vi "New motor Control integrated remodeled PID revisit.vi"(0 "States":enum16{"RESET ENCODER", "WRITE", "READ", "INIT"}(ring), 1 "Target Speed":T2 {"wTargetSpeed" scale=-1.0..1.0; "yTargetSpeed" scale=-1.0..1.0; "xTargetSpeed" scale=-1.0..1.0}, 3 "Error in":errorcluster, 4 "Boolean":bool=TRUE) -> (5 "Speed and distance cluster":T1, 6 "Error out":errorcluster)   [LabVIEW 2018]
uses:
  <vilib>/addons/control/pid/pid.llb/PID (DBL).vi
  <vilib>/addons/control/pid/NI_PID_pid.lvlib
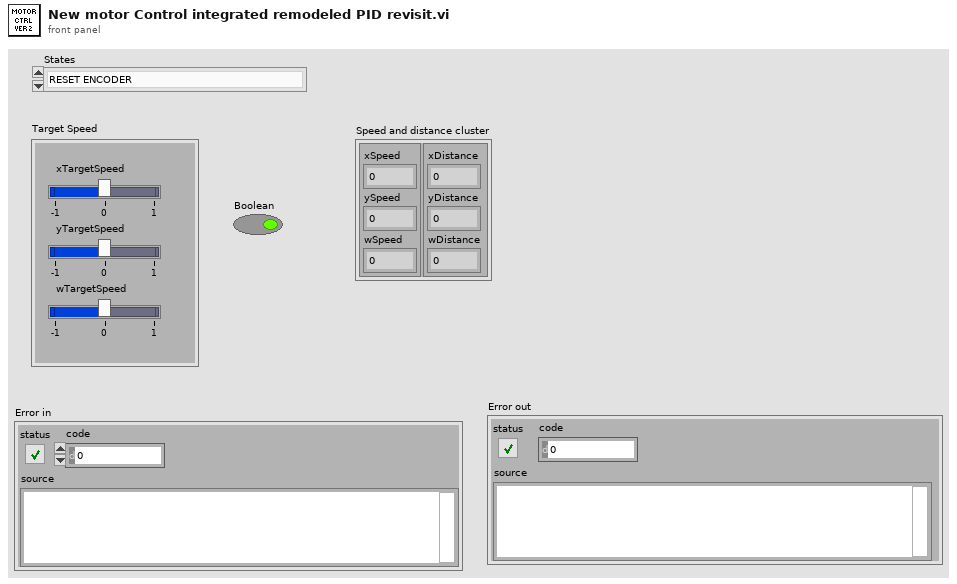
[diagram p1: front panel]
types:
  T1 = cluster{cluster{"xSpeed":dbl, "ySpeed":dbl, "wSpeed":dbl}, cluster{"xDistance":dbl, "yDistance":dbl, "wDistance":dbl}}
  T2 = cluster{"xTargetSpeed":dbl, "yTargetSpeed":dbl, "wTargetSpeed":dbl}
  T3 = cluster{"Encoder 0":dbl, "Encoder 1":dbl, "Encoder 2":dbl}
  T4 = cluster{"proportional gain (Kc)":dbl, "integral time (Ti, min)":dbl, "derivative time (Td, min)":dbl}
  T5 = cluster{"Distance M0 ":dbl, "Distance M1 ":dbl, "Distance M2 ":dbl}
  T6 = cluster{"xDistance":dbl, "yDistance":dbl, "wDistance":dbl}
  T7 = cluster{"xSpeed":dbl, "ySpeed":dbl, "wSpeed":dbl}
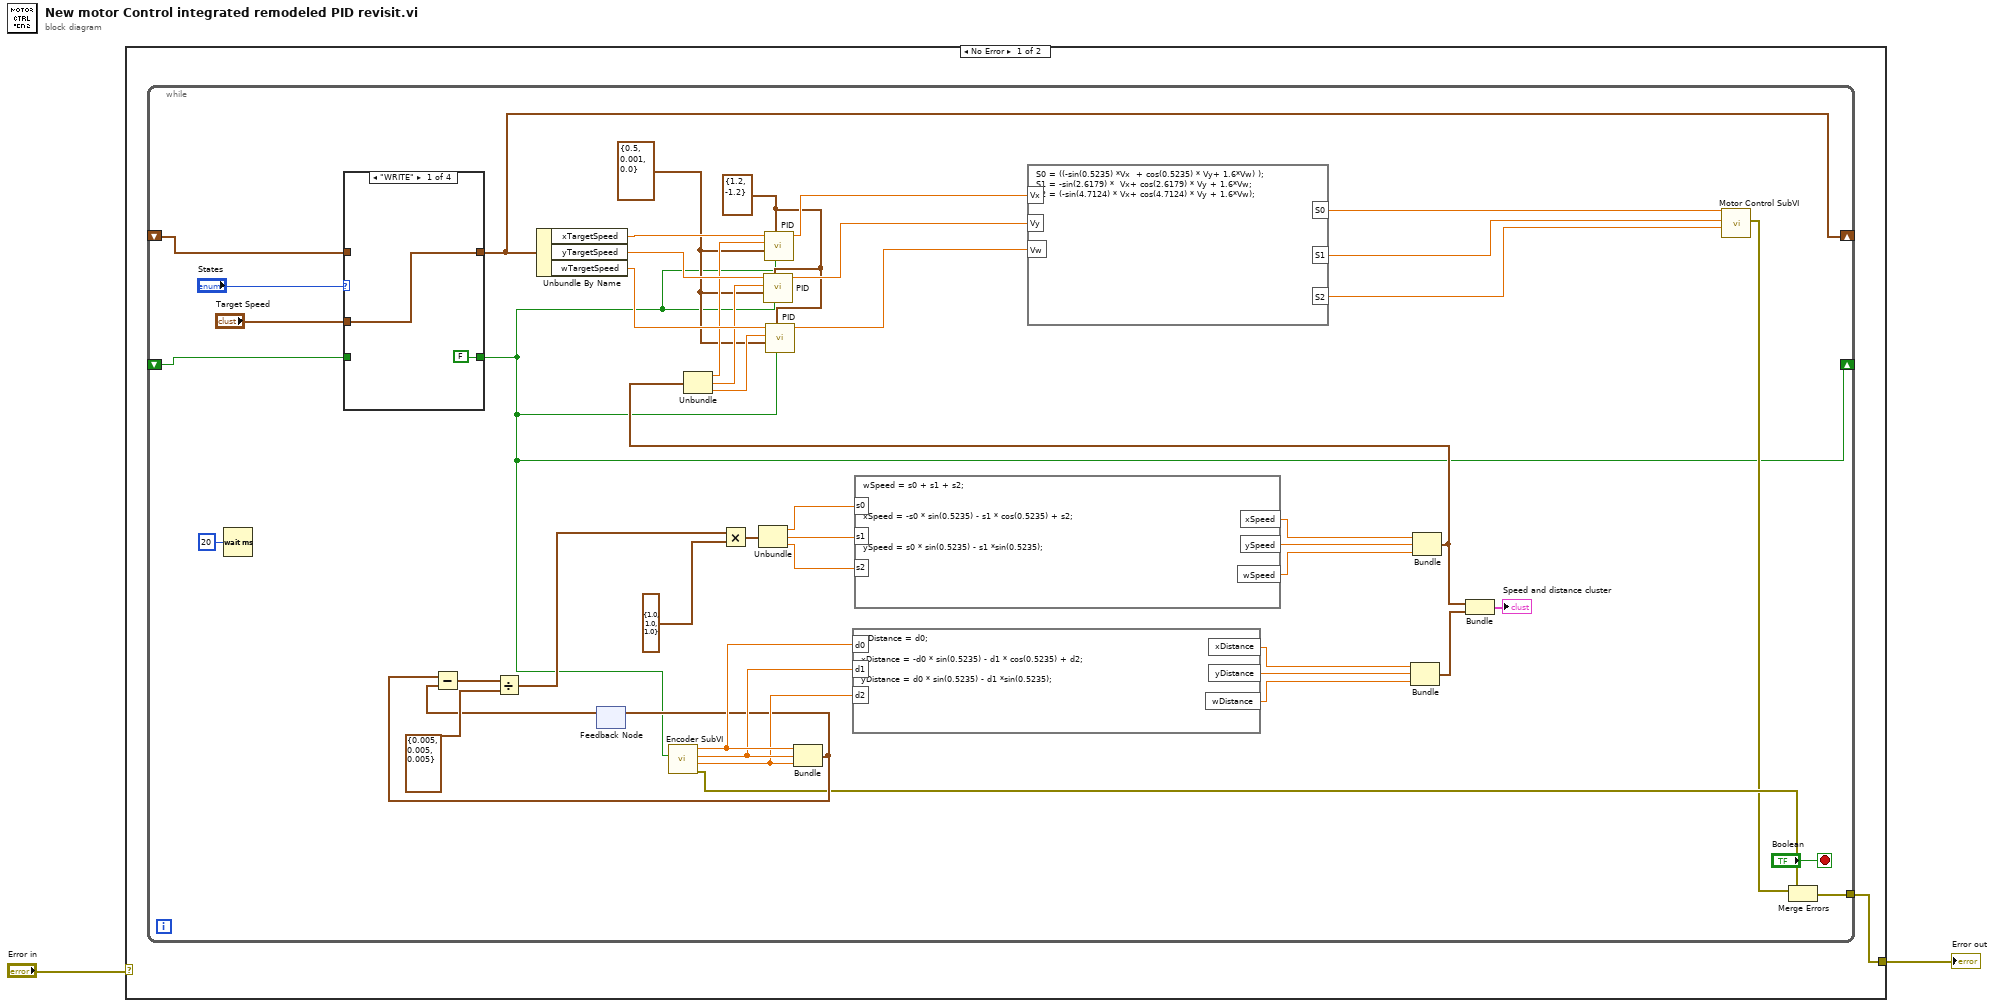
[diagram p0: block diagram]
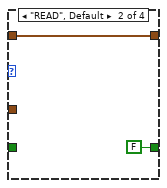
[diagram p2: hidden frame]
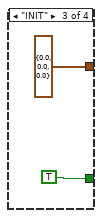
[diagram p3: hidden frame]
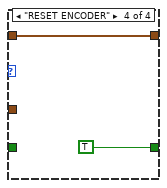
[diagram p4: hidden frame]
diagram:
  n1 = case shown="No Error" "Error in" {
    selector: "Error in" -> [_ w59]
    tunnel: [w3 w59] -> w1
    frame No Error {
      n2 = while {
        shift-right: [w29] -> _
        shift-left: _ -> [w28]
        tunnel: [w23] -> w3
        shift-right: [w5] -> _
        shift-left: _ -> [w22]
        stop <- "Boolean" stop-if-true
        w6 = T4 {"proportional gain (Kc)"=0.5, "integral time (Ti, min)"=0.001, "derivative time (Td, min)"=0.0} ("PID gains")
        w7 = cluster{"output high":dbl, "output low":dbl} {"output high"=1.2, "output low"=-1.2} ("output range")
        n3 = Wait (ms)(milliseconds to wait=u32 20) -> ()  [unwired: 1 out]
        n4 = case shown="\"WRITE\"" "States" {
          tunnel: "Target Speed" -> [w52 _ _ _]
          tunnel: [w52 w54 T2 {"xTargetSpeed"=0.0, "yTargetSpeed"=0.0, "wTargetSpeed"=0.0} ("Target Speed") w58] -> w29
          tunnel: w28 -> [_ w54 _ w58]
          tunnel: [FALSE ("Reset Encoders") FALSE ("Reset Encoders") TRUE TRUE ("Reset Encoders")] -> w5
          tunnel: w22 -> [_ _ _ _]
          frame "WRITE" {
          }
          frame "READ", Default {
          }
          frame "INIT" {
          }
          frame "RESET ENCODER" {
          }
        }
        n5 = Unbundle By Name(w29) -> ("xTargetSpeed"=w17:dbl, "yTargetSpeed"=w16:dbl, "wTargetSpeed"=w15:dbl)
        n6 = feedback #1() -> (w43:T5)  [unwired: 1 in]
        n7 = call "Encoder SubVI.vi"("Reset Encoders"=w5) -> ("error out"=w25:errorcluster, "Distance M2"=w40:dbl, "Distance M1"=w41:dbl, "Distance M0"=w42:dbl)  [unwired: 7 in]
        n8 = Bundle("Distance M0"=w42, "Distance M1"=w41, "Distance M2"=w40) -> (w32:T5)  [unwired: 1 in]
        n9 = Subtract(x=w32, y=w43) -> (x-y=w50:T5)
        n10 = Divide(x=w50, y=T3 {"Encoder 0"=0.005, "Encoder 1"=0.005, "Encoder 2"=0.005}) -> (x/y=w36:cluster{dbl, dbl, dbl})
        n11 = feedback-in #1(w32) -> ()
        n12 = Multiply(x=w36, y=cluster{dbl, dbl, dbl} {1.0, 1.0, 1.0}) -> (x*y=w21:cluster{dbl, dbl, dbl})
        n13 = Unbundle(w21) -> (w34:dbl, w45:dbl, w44:dbl)
        n14 = formula code="wDistance = d0;\n\nxDistance = -d0 * sin(0.5235) - d1 * cos(0.5235) + d2;\n\nyDistance = d0 * sin(0.5235) - d1 *sin(0.5235);"("d0"=w42, "d1"=w41, "d2"=w40) -> ("xDistance"=w39:dbl, "wDistance"=w37:dbl, "yDistance"=w38:dbl)
        n15 = formula code="wSpeed = s0 + s1 + s2;\n\n\nxSpeed = -s0 * sin(0.5235) - s1 * cos(0.5235) + s2;\n\n\nySpeed = s0 * sin(0.5235) - s1 *sin(0.5235);"("s0"=w34, "s1"=w45, "s2"=w44) -> ("xSpeed"=w47:dbl, "ySpeed"=w48:dbl, "wSpeed"=w46:dbl)
        n16 = Bundle("xDistance"=w39, "yDistance"=w38, "wDistance"=w37) -> (w27:T6)  [unwired: 1 in]
        n17 = Bundle("xSpeed"=w47, "ySpeed"=w48, "wSpeed"=w46) -> (w11:T7)  [unwired: 1 in]
        n18 = Unbundle(w11) -> ("xSpeed"=w10:dbl, "ySpeed"=w9:dbl, "wSpeed"=w8:dbl)
        n19 = call-poly <vilib>:"PID.vi"("reinitialize? (F)"=w5, "output range"=w7, "PID gains"=w6, "process variable"=w9, "setpoint"=w16) -> ("output"=w13:dbl)  [unwired: 5 in, 1 out]
        n20 = call-poly <vilib>:"PID.vi"("reinitialize? (F)"=w5, "output range"=w7, "PID gains"=w6, "process variable"=w10, "setpoint"=w17) -> ("output"=w14:dbl)  [unwired: 5 in, 1 out]
        n21 = call-poly <vilib>:"PID.vi"("reinitialize? (F)"=w5, "output range"=w7, "PID gains"=w6, "process variable"=w8, "setpoint"=w15) -> ("output"=w12:dbl)  [unwired: 5 in, 1 out]
        n22 = formula code="S0 = ((-sin(0.5235) *Vx  + cos(0.5235) * Vy+ 1.6*Vw) );\nS1 = -sin(2.6179) *  Vx+ cos(2.6179) * Vy + 1.6*Vw;\nS2 = (-sin(4.7124) * Vx+ cos(4.7124) * Vy + 1.6*Vw);"("Vx"=w14, "Vy"=w13, "Vw"=w12) -> ("S0"=w20:dbl, "S1"=w19:dbl, "S2"=w18:dbl)
        n23 = Bundle(w11, w27) -> (→"Speed and distance cluster":T1)  [unwired: 1 in]
        n24 = call "Motor Control SubVI.vi"("Speed M2"=w18, "Speed M1"=w19, "Speed M0"=w20) -> ("Motor Error"=w24:errorcluster)  [unwired: 8 in]
        n25 = Merge Errors(w24, w25) -> (w23:errorcluster)
      }
    }
    frame Error {
    }
  }
  "Error out" <- w1
